vi "IMAQ flattened string to array.vi"(11 "Flattened Image String":string) -> (3 "Image Pixels (U16)":u16[][](array[numeric]))   [LabVIEW 2020]
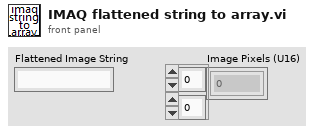
[diagram p1: front panel]
types:
  T1 = typedef "Image Type" = u32
  T2 = typedef "IMAQ Image.ctl" = refnum<image>
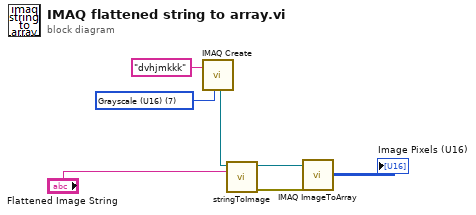
[diagram p0: block diagram]
diagram:
  w3 = T1 7 items=["Grayscale (U8)", "Grayscale (I16)", "Grayscale (SGL)", "Complex (CSG)", "RGB (U32)", "HSL (U32)", "RGB (U64)", "Grayscale (U16)"] ("Image Type")
  n1 = call "IMAQ Create"("Image Name"="dvhjmkkk", "Image Type"=w3) -> ("New Image"=w4:T2)  [unwired: 3 in, 1 out]
  n2 = call "stringToImage.vi"("data in"="Flattened Image String", "Refnum in"=w4) -> ("error out"=w7:errorcluster, "Refnum out"=w5:T2)  [unwired: 6 in, 2 out]
  n3 = call "IMAQ ImageToArray"("error in (no error)"=w7, "Image"=w5) -> ("Image Pixels (U16)"=→"Image Pixels (U16)":u16[][])  [unwired: 2 in, 4 out]
